vi "AttackerStopRole.vi"(8 "error in (no error)":errorcluster, 10 "Game in":refnum<class "Game.lvclass">, 11 "AttackerStopRole in":refnum<class "AttackerStopRole.lvclass">) -> (0 "error out":errorcluster, 1 "Numeric":i32, 2 "Robot out":refnum<class "Robot.lvclass">, 3 "AttackerStopRole out":refnum<class "AttackerStopRole.lvclass">)   [LabVIEW 2018, in "AttackerStopRole.lvclass"]
uses:
  AttackerStopRole.lvclass
  C:/Users/anton/Desktop/roboime/PS 2020.1/SSL_AI/Role_class/Role.lvclass
  Game_class/Game.lvclass
  Robot_class/Robot.lvclass
  Role_class/Role.lvclass/Role.ctl
  AttackerStopTactic_class/States.ctl
  Tacticbook_class/Tacticbook.lvclass/Tacticbook.ctl
  HaltTactic_class/HaltTactic.lvclass/HaltTactic.ctl
  Tacticbook_class/Read HaltTactic.vi
  HaltTactic_class/Read States.vi
  Tacticbook_class/Write HaltTactic.vi
  Role_class/Read Tacticbook.vi
  Role_class/Read tactic_index.vi
  Role_class/Write Tacticbook.vi
  Role_class/Write tactic_index.vi
  Role_class/Read RobotRef.vi
  Tacticbook_class/Tacticbook.lvclass
  HaltTactic_class/HaltTactic.lvclass
  AttackerStopTactic_class/AttackerStopTactic.lvclass
panel:
  out "Game out":refnum<class "Game.lvclass">
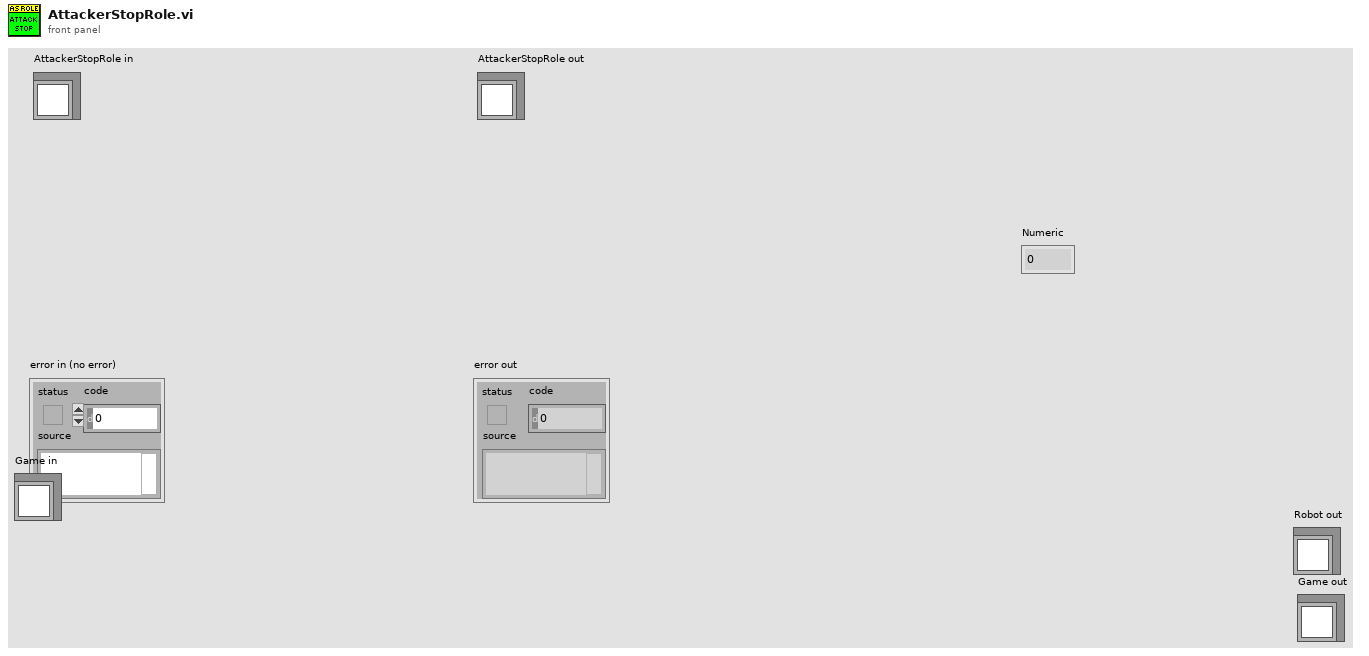
[diagram p1: front panel]
types:
  T1 = typedef "AttackerStopTactic.lvclass/States.ctl" = enum16{"Block", "AimGoal", "Exit"}
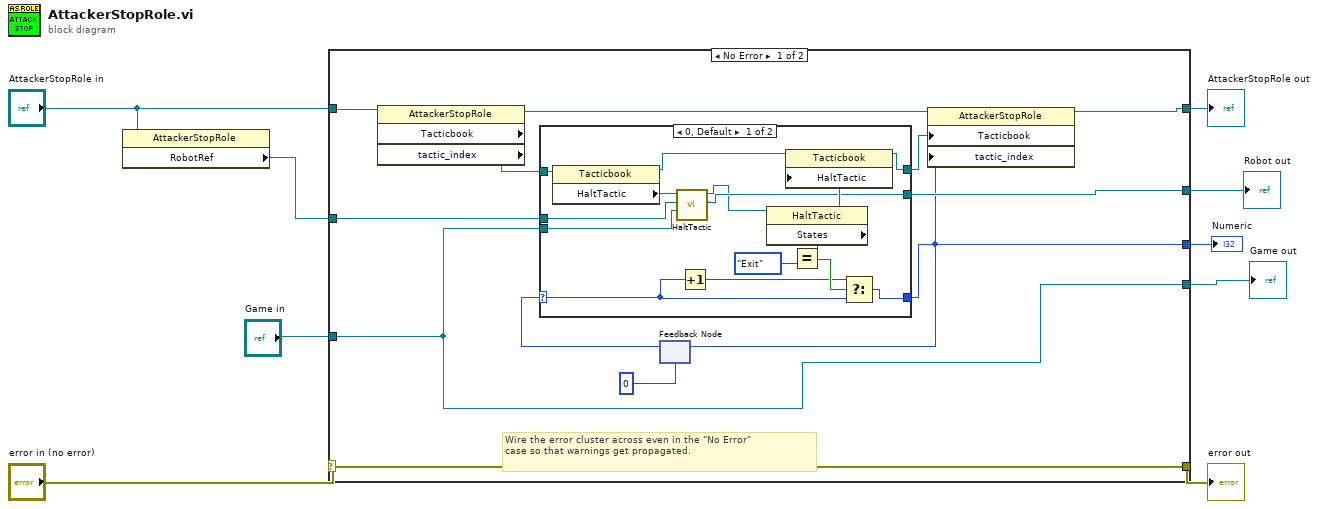
[diagram p0: block diagram]
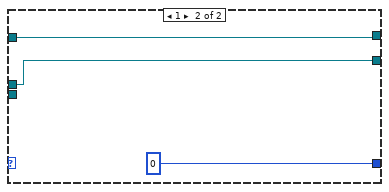
[diagram p2: hidden frame]
diagram:
  n1 = property class="AttackerStopRole"(reference="AttackerStopRole in") -> ("RobotRef"=w4:refnum<class "Robot.lvclass">)  [unwired: 1 in, 2 out]
  n2 = case shown="No Error" "error in (no error)" {
    selector: "error in (no error)" -> [w21 w43]
    tunnel: [w21 w43] -> w8
    tunnel: [w14 w42] -> w7
    tunnel: "AttackerStopRole in" -> [w15 w42]
    tunnel: "Game in" -> [w12 w40]
    tunnel: w4 -> [w13 w41]
    tunnel: [w12 w40] -> w3
    tunnel: [w11 w41] -> w2
    tunnel: [w10 _] -> w1
    frame No Error {
      # "Wire the error cluster across even in the \"No Error\"\ncase so that warnings get propagated."
      n3 = property class="AttackerStopRole" props=["Tacticbook", "tactic_index"](reference=w15) -> (reference out=w20:refnum<class "AttackerStopRole.lvclass">, "Tacticbook"=w17:refnum<class "Tacticbook.lvclass">)  [unwired: 1 in, 2 out]
      n4 = feedback #1(0) -> (w18:i32)
      n5 = case shown="0, Default" w18 {
        selector: w18 -> [w32 _]
        tunnel: [w33 0] -> w10
        tunnel: w17 -> [w36 w37]
        tunnel: w13 -> [w25 w39]
        tunnel: [w23 w39] -> w11
        tunnel: [w28 w37] -> w16
        tunnel: w12 -> [w24 _]
        frame 0, Default {
          n6 = property class="Tacticbook"(reference=w36) -> (reference out=w30:refnum<class "Tacticbook.lvclass">, "HaltTactic"=w26:refnum<class "HaltTactic.lvclass">)  [unwired: 1 in, 1 out]
          n7 = call-dynamic "HaltTactic.vi"("Game in"=w24, "Robot"=w25, "HaltTactic in"=w26) -> ("Robot out"=w23:refnum<class "Robot.lvclass">, "HaltTactic out"=w22:refnum<class "HaltTactic.lvclass">)  [unwired: 6 in, 1 out]
          n8 = Increment(x=w32) -> (x+1=w31:i32)
          n9 = property class="HaltTactic"(reference=w22) -> (reference out=w29:refnum<class "HaltTactic.lvclass">, "States"=w35:enum16{"Halt", "Exit"})  [unwired: 1 in, 1 out]
          n10 = property class="Tacticbook"(reference=w30, "HaltTactic"=w29) -> (reference out=w28:refnum<class "Tacticbook.lvclass">)  [unwired: 1 in, 1 out]
          n11 = Equal?(x=w35, y=States."Exit") -> (x = y?=w34:bool)
          n12 = Select(t=w31, s=w34, f=w32) -> (s? t:f=w33:i32)
        }
        frame 1 {
        }
      }
      n13 = feedback-in #1(w10) -> ()
      n14 = property class="AttackerStopRole"(reference=w20, "Tacticbook"=w16, "tactic_index"=w10) -> (reference out=w14:refnum<class "AttackerStopRole.lvclass">)  [unwired: 1 in, 1 out]
    }
    frame Error {
    }
  }
  "error out" <- w8
  "AttackerStopRole out" <- w7
  "Robot out" <- w2
  "Game out" <- w3
  "Numeric" <- w1
